vi "chr63204A_Mode_selector.vi"(8 "error in (no error)":errorcluster, 9 "Mode":T1(ring), 10 "Level":enum16{"Z", "L", "M", "H"}(ring), 11 "VISA resource name":refnum<visa-resource-name>) -> (0 "error out":errorcluster, 3 "VISA resource name out":refnum<visa-resource-name>)   [LabVIEW 2020]
doc: "More user-friendly version of mode selector for chroma 63204A"
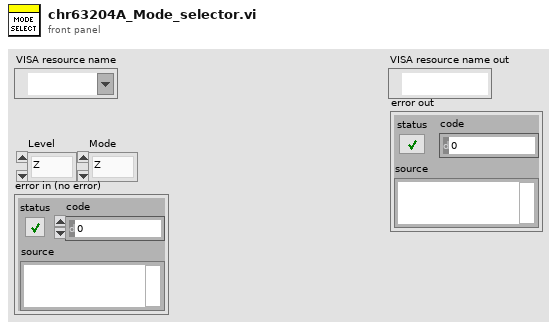
[diagram p1: front panel]
types:
  T1 = enum16{"Z", "CC", "CR", "CV", "CP", "CCD", "CRD", "BAT", "SWD", "OCP", "CCS", "CZ", "CVCC", "CRCC", "CVCR", "AUTO", "PROG", "UDW", "EXT"}
  T2 = enum16{"CCL", "CCM", "CCH", "CRL", "CRM", "CRH", "CVL", "CVM", "CVH", "CPL", "CPM", "CPH", "CCDL", "CCDM", "CCDH", "CRDL", "CRDM", "CRDH", "BATL", "BATM", "BATH", "SWDL", "SWDM", "SWDH", "OCPL", "OCPM", "OCPH", "CCSL", "CCSM", "CCSH", "CZL", "CZM", "CZH", "CVCC", "CRCC", "CVCR", "AUTO", "PROG", "UDWL", "UDWM", "UDWH", "EXTL", "EXTM", "EXTH"}
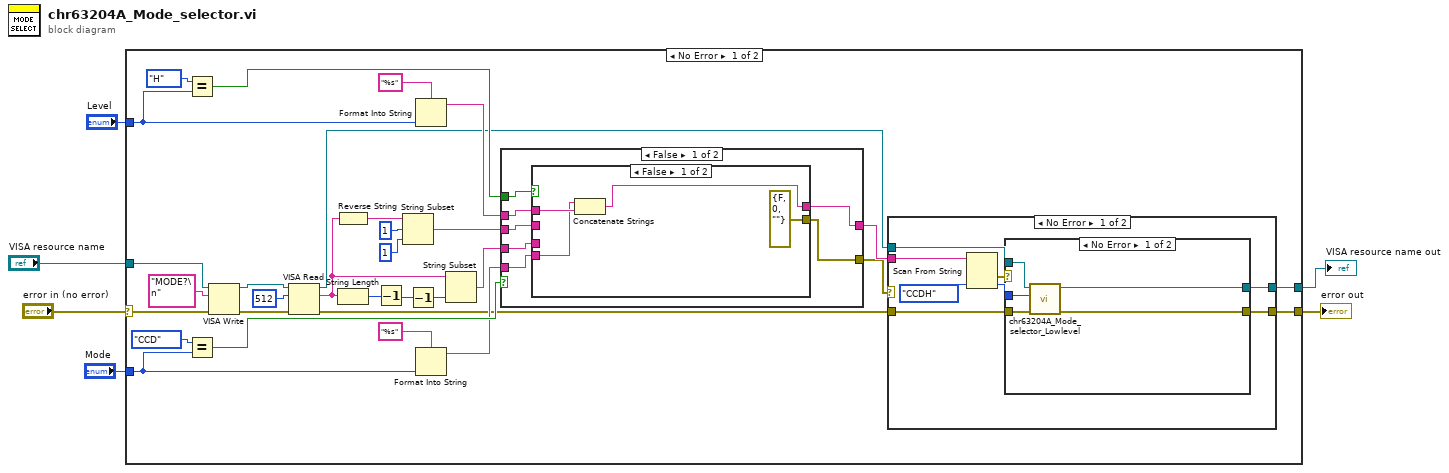
[diagram p0: block diagram]
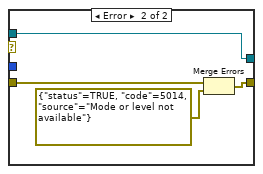
[diagram p2: hidden frame]
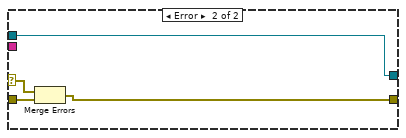
[diagram p3: hidden frame]
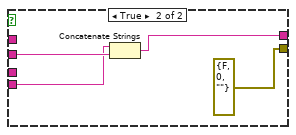
[diagram p4: hidden frame]
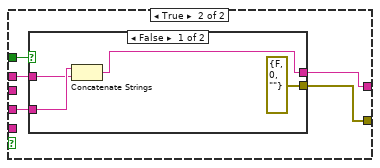
[diagram p5: hidden frame]
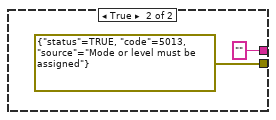
[diagram p6: hidden frame]
diagram:
  n1 = case shown="No Error" "error in (no error)" {
    selector: "error in (no error)" -> [w11 w85]
    tunnel: "Level" -> [w22 _]
    tunnel: "Mode" -> [w19 _]
    tunnel: "VISA resource name" -> [w12 w86]
    tunnel: [w10 w86] -> w2
    tunnel: [w9 w85] -> w1
    frame No Error {
      n2 = Equal?(x=enum16{"Z", "L", "M", "H"}."H" ("Level 2"), y=w22) -> (x = y?=w36:bool)
      n3 = Equal?(x=T1."CCD" ("Mode 3"), y=w19) -> (x = y?=w37:bool)
      n4 = VISA Write(VISA resource name=w12, write buffer="MODE?\n", error in (no error)=w11) -> (VISA resource name out=w33:refnum<visa-resource-name>, error out=w32:errorcluster)  [unwired: 1 out]
      n5 = VISA Read(VISA resource name=w33, byte count=u32 512, error in (no error)=w32) -> (VISA resource name out=w14:refnum<visa-resource-name>, read buffer=w27:string, error out=w13:errorcluster)  [unwired: 1 out]
      n6 = Reverse String(1:w27) -> (0:w29:string)
      n7 = String Length(string=w27) -> (length=w28:i32)
      n8 = Decrement(x=w28) -> (x-1=w8:i32)
      n9 = String Subset(string=w29, offset (0)=1, length (rest)=1 ("length (rest)")) -> (substring=w26:string)
      n10 = Decrement(x=w8) -> (x-1=w7:i32)
      n11 = Format Into String(format string="%s", w22) -> (resulting string=w17:string)  [unwired: 2 in, 1 out]
      n12 = Format Into String(format string="%s", w19) -> (resulting string=w18:string)  [unwired: 2 in, 1 out]
      n13 = String Subset(string=w27, length (rest)=w7) -> (substring=w25:string)  [unwired: 1 in]
      n14 = case shown="False" w37 {
        tunnel: w36 -> [w65 w78]
        tunnel: w26 -> [w64 _]
        tunnel: w25 -> [w62 w74]
        tunnel: [w61 w77] -> w15
        tunnel: w18 -> [w63 _]
        tunnel: w17 -> [w59 w76]
        tunnel: [w60 w75] -> w16
        frame False {
          n15 = case shown="False" w65 {
            tunnel: [errorcluster {"status"=FALSE, "code"=0, "source"=""} ("error constant") errorcluster {"status"=FALSE, "code"=0, "source"=""} ("error constant")] -> w61
            tunnel: w62 -> [_ _]
            tunnel: [w69 w70] -> w60
            tunnel: w64 -> [_ w73]
            tunnel: w63 -> [w66 w72]
            tunnel: w59 -> [w67 _]
            frame False {
              n16 = Concatenate Strings(w66, w67) -> (w69:string)
            }
            frame True {
              n17 = Concatenate Strings(w72, w73) -> (w70:string)
            }
          }
        }
        frame True {
          n18 = case shown="False" w78 {
            tunnel: [errorcluster {"status"=FALSE, "code"=0, "source"=""} ("error constant") errorcluster {"status"=TRUE, "code"=5013, "source"="Mode or level must be assigned"} ("error constant")] -> w77
            tunnel: w74 -> [w82 _]
            tunnel: w76 -> [w81 _]
            tunnel: [w80 ""] -> w75
            frame False {
              n19 = Concatenate Strings(w82, w81) -> (w80:string)
            }
            frame True {
            }
          }
        }
      }
      n20 = case shown="No Error" w15 {
        selector: w15 -> [_ w58]
        tunnel: w16 -> [w44 _]
        tunnel: w14 -> [w42 w57]
        tunnel: w13 -> [w41 w55]
        tunnel: [w39 w57] -> w10
        tunnel: [w38 w56] -> w9
        frame No Error {
          n21 = Scan From String(input string=w44, default 1=T2."CCDH" ("Mode")) -> (error out=w43:errorcluster, output 1=w40:T2)  [unwired: 3 in, 2 out]
          n22 = case shown="No Error" w43 {
            tunnel: [w47 w53] -> w38
            tunnel: w42 -> [w50 w51]
            tunnel: w41 -> [w49 w54]
            tunnel: w40 -> [w48 _]
            tunnel: [w46 w51] -> w39
            frame No Error {
              n23 = call "chr63204A_Mode_selector_Lowlevel.vi"("error in (no error)"=w49, "Mode"=w48, "VISA resource name"=w50) -> ("error out"=w47:errorcluster, "VISA resource name out"=w46:refnum<visa-resource-name>)  [unwired: 7 in]
            }
            frame Error {
              n24 = Merge Errors(w54, errorcluster {"status"=TRUE, "code"=5014, "source"="Mode or level not available"} ("error constant")) -> (w53:errorcluster)
            }
          }
        }
        frame Error {
          n25 = Merge Errors(w58, w55) -> (w56:errorcluster)
        }
      }
    }
    frame Error {
    }
  }
  "VISA resource name out" <- w2
  "error out" <- w1
